vi "Start Measurement.vi"(8 "error in (no error)":errorcluster, 10 "Launch Measurements Message in":refnum<class "Launch Measurements Message.lvclass">, 11 "Controller in":refnum<class "Controller.lvclass">) -> (0 "error out":errorcluster, 3 "Controller out":refnum<class "Controller.lvclass">)   [LabVIEW 2016, in "Controller Actor.lvlib" / "Controller.lvclass"]
uses:
  Controller.lvclass
  C:/Program Files (x86)/National Instruments/LabVIEW 2016/vi.lib/ActorFramework/Actor/Actor.lvclass
  Messages/Launch Measurements Message/Launch Measurements Message.lvclass
  Messages/Launch Measurements Message/Launch Measurements Message.lvclass/Launch Measurements Message.ctl
  Measurement Actor/Measurement.lvclass/Measurement.ctl
  <vilib>/ActorFramework/Actor/Actor.lvclass/Actor.ctl
  <vilib>/ActorFramework/Message Enqueuer/Message Enqueuer.lvclass/Message Enqueuer.ctl
  Measurement Actor/Accessors/Write Time Measurement Requested.vi
  Measurement Actor/Write GUID.vi
  Measurement Actor/Accessors/Write Continuous Run.vi
  Messages/Launch Measurements Message/Read Measurement Name.vi
  Messages/Launch Measurements Message/Read Device Names.vi
  Messages/Launch Measurements Message/Read Show FP_.vi
  Messages/Launch Measurements Message/Read Time Measurement Requested 2.vi
  Messages/Launch Measurements Message/Read GUID.vi
  Messages/Launch Measurements Message/Read Continuous Run 2.vi
  <vilib>/ActorFramework/Message Enqueuer/Init from Existing Queue.vi
  Measurement Actor/Measurement.lvclass
  Measurement Actor/Properties/Write Array of Hardware 2.vi
  Measurement Actor/Properties/Write Show UI While Running 2.vi
  <vilib>/ActorFramework/Message Enqueuer/Message Enqueuer.lvclass
  <vilib>/ActorFramework/Actor/Actor.lvclass
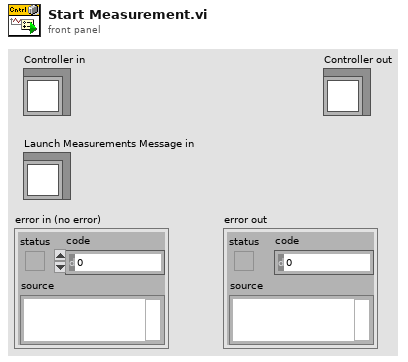
[diagram p1: front panel]
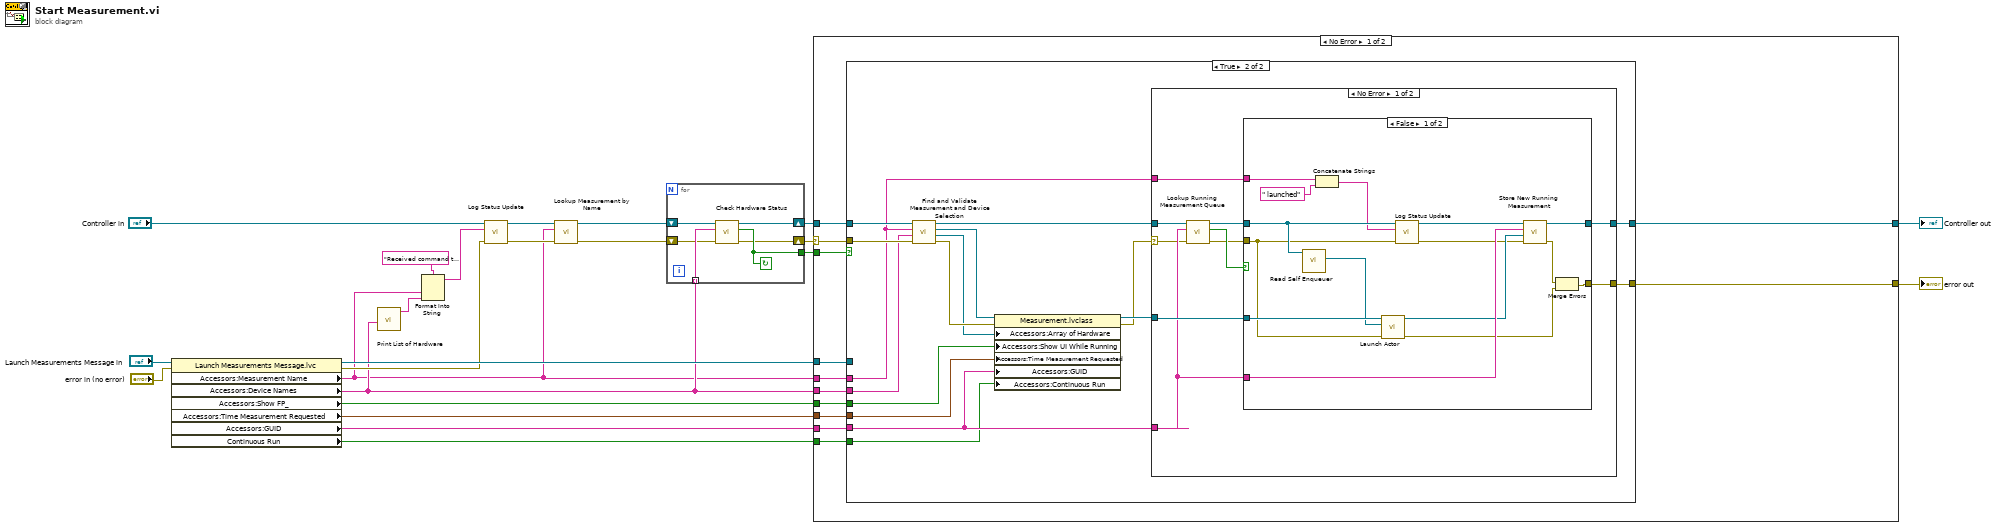
[diagram p0: block diagram]
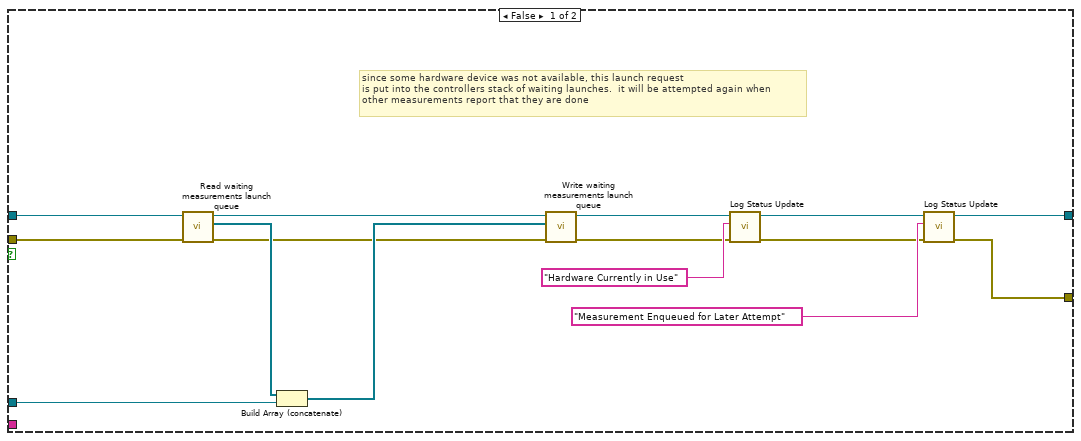
[diagram p2: hidden frame]
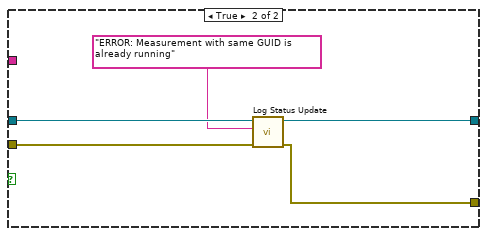
[diagram p3: hidden frame]
diagram:
  n1 = property class="Launch Measurements Message.lvc"(reference="Launch Measurements Message in", error in="error in (no error)") -> (reference out=w13:refnum<class "Launch Measurements Message.lvclass">, error out=w8:errorcluster, "Accessors:Measurement Name"=w2:string, "Accessors:Device Names"=w7:string[], "Accessors:Show FP_"=w10:bool, "Accessors:Time Measurement Requested"=w9:timestamp, "Accessors:GUID"=w12:string, "Continuous Run"=w1:bool)
  n2 = call "Print List of Hardware.vi"("Device Names"=w7) -> ("String"=w22:string)  [unwired: 10 in]
  n3 = Format Into String(format string="Received command to run %s using %s", w2, w22) -> (resulting string=w21:string)  [unwired: 2 in, 1 out]
  n4 = call-dynamic "Log Status Update.vi"("error in (no error)"=w8, "String"=w21, "Controller in"="Controller in") -> ("error out"=w5:errorcluster, "Controller out"=w6:refnum<class "Controller.lvclass">)  [unwired: 7 in]
  n5 = call "Lookup Measurement by Name.vi"("error in (no error)"=w5, "Measurement Name"=w2, "Controller in"=w6) -> ("error out"=w4:errorcluster, "Controller out"=w3:refnum<class "Controller.lvclass">)  [unwired: 5 in, 2 out]
  n6 = for {
    shift-right: [w28] -> w18
    shift-left: w3 -> [w29]
    tunnel: w7 -> [w27] mode=indexing
    tunnel: [w26] -> w19
    shift-right: [w25] -> w17
    shift-left: w4 -> [w24]
    stop <- w26 continue-if-true
    n7 = call "Check Hardware Status.vi"("error in (no error)"=w24, "Device Name"=w27, "Controller in"=w29) -> ("error out"=w25:errorcluster, "Available?"=w26:bool, "Controller out"=w28:refnum<class "Controller.lvclass">)  [unwired: 6 in]
  }
  n8 = case shown="No Error" w17 {
    selector: w17 -> [w32 w106]
    tunnel: w19 -> [w41 _]
    tunnel: w18 -> [w33 w105]
    tunnel: [w40 w105] -> w15
    tunnel: w12 -> [w39 _]
    tunnel: [w38 w106] -> w14
    tunnel: w13 -> [w37 _]
    tunnel: w10 -> [w36 _]
    tunnel: w9 -> [w35 _]
    tunnel: w2 -> [w34 _]
    tunnel: w7 -> [w31 _]
    tunnel: w1 -> [w30 _]
    frame No Error {
      n9 = case shown="True" w41 {
        tunnel: [w43 w72] -> w40
        tunnel: w33 -> [w54 w70]
        tunnel: w32 -> [w52 w69]
        tunnel: [w44 w68] -> w38
        tunnel: w39 -> [_ w60]
        tunnel: w37 -> [w42 _]
        tunnel: w36 -> [_ w58]
        tunnel: w35 -> [_ w59]
        tunnel: w34 -> [_ w61]
        tunnel: w31 -> [_ w62]
        tunnel: w30 -> [_ w57]
        frame False {
          # "since some hardware device was not available, this launch request\nis put into the controllers stack of waiting launches.  it will be attempted again when\nother measurements report that they are done"
          n10 = call "Read waiting measurements launch queue.vi"("error in (no error)"=w52, "Controller in"=w54) -> ("error out"=w51:errorcluster, "stack of waiting msmt requests"=w56:refnum<class "Launch Measurements Message.lvclass">[], "Controller out"=w55:refnum<class "Controller.lvclass">)  [unwired: 7 in]
          n11 = Build Array (concatenate)(w56, w42) -> (w53:refnum<class "Launch Measurements Message.lvclass">[])
          n12 = call "Write waiting measurements launch queue.vi"("error in (no error)"=w51, "stack of waiting msmt requests"=w53, "Controller in"=w55) -> ("error out"=w46:errorcluster, "Controller out"=w47:refnum<class "Controller.lvclass">)  [unwired: 7 in]
          n13 = call-dynamic "Log Status Update.vi"("error in (no error)"=w46, "String"="Hardware Currently in Use", "Controller in"=w47) -> ("error out"=w45:errorcluster, "Controller out"=w48:refnum<class "Controller.lvclass">)  [unwired: 7 in]
          n14 = call-dynamic "Log Status Update.vi"("error in (no error)"=w45, "String"="Measurement Enqueued for Later Attempt", "Controller in"=w48) -> ("error out"=w44:errorcluster, "Controller out"=w43:refnum<class "Controller.lvclass">)  [unwired: 7 in]
        }
        frame True {
          n15 = call "Find and Validate Measurement and Device Selection.vi"("error in (no error)"=w69, "Device Names"=w62, "Measurement Name"=w61, "Controller in"=w70) -> ("error out"=w66:errorcluster, "Hardware Objects"=w65:refnum<class "Hardware.lvclass">[], "Measurement out"=w64:refnum<class "Measurement.lvclass">, "Controller out"=w67:refnum<class "Controller.lvclass">)  [unwired: 4 in]
          n16 = property class="Measurement.lvclass"(reference=w64, error in=w66, "Accessors:Array of Hardware"=w65, "Accessors:Show UI While Running"=w58, "Accessors:Time Measurement Requested"=w59, "Accessors:GUID"=w60, "Accessors:Continuous Run"=w57) -> (reference out=w71:refnum<class "Measurement.lvclass">, error out=w63:errorcluster)
          n17 = case shown="No Error" w63 {
            selector: w63 -> [w74 w104]
            tunnel: [w82 w103] -> w72
            tunnel: w71 -> [w78 _]
            tunnel: w67 -> [w77 w103]
            tunnel: w60 -> [w76 _]
            tunnel: [w75 w104] -> w68
            tunnel: w61 -> [w73 _]
            frame No Error {
              n18 = call "Lookup Running Measurement Queue.vi"("error in (no error)"=w74, "Measurement Name.Harware()"=w76, "Controller in"=w77) -> ("error out"=w79:errorcluster, "Found?"=w80:bool, "Controller out"=w81:refnum<class "Controller.lvclass">)  [unwired: 5 in, 1 out]
              n19 = case shown="False" w80 {
                tunnel: [w97 w101] -> w82
                tunnel: w78 -> [w96 _]
                tunnel: w76 -> [w95 _]
                tunnel: w81 -> [w93 w102]
                tunnel: w79 -> [w87 w99]
                tunnel: [w84 w98] -> w75
                tunnel: w73 -> [w83 _]
                frame False {
                  n20 = call <vilib>:"Read Self Enqueuer.vi"("Actor"=w93) -> ("Self Enqueuer"=w92:refnum<class "Message Enqueuer.lvclass">)  [unwired: 10 in]
                  n21 = Concatenate Strings(w83, " launched" ("string")) -> (w89:string)
                  n22 = call <vilib>:"Launch Actor.vi"("error in (no error)"=w87, "Actor-to-Caller Enqueuer"=w92, "Actor"=w96) -> ("error out"=w85:errorcluster, "Caller-To-Actor Enqueuer"=w91:refnum<class "Message Enqueuer.lvclass">)  [unwired: 7 in]
                  n23 = call-dynamic "Log Status Update.vi"("error in (no error)"=w87, "String"=w89, "Controller in"=w93) -> ("error out"=w88:errorcluster, "Controller out"=w90:refnum<class "Controller.lvclass">)  [unwired: 7 in]
                  n24 = call "Store New Running Measurement.vi"("error in (no error)"=w88, "Caller-To-Actor Enqueuer"=w91, "name"=w95, "Controller in"=w90) -> ("error out"=w86:errorcluster, "Controller out"=w97:refnum<class "Controller.lvclass">)  [unwired: 6 in]
                  n25 = Merge Errors(w86, w85) -> (w84:errorcluster)
                }
                frame True {
                  n26 = call-dynamic "Log Status Update.vi"("error in (no error)"=w99, "String"="ERROR: Measurement with same GUID is already running", "Controller in"=w102) -> ("error out"=w98:errorcluster, "Controller out"=w101:refnum<class "Controller.lvclass">)  [unwired: 7 in]
                }
              }
            }
            frame Error {
            }
          }
        }
      }
    }
    frame Error {
    }
  }
  "error out" <- w14
  "Controller out" <- w15
